vi "Autoliftswitch.vi"() -> ()   [LabVIEW 2017]
uses:
  <vilib>/Rock Robotics/WPI/ThirdParty/Phoenix-LabVIEW/Motor Controller/Controls/CTRE_Phoenix_MotorControl_ControlMode.ctl
  <vilib>/Rock Robotics/WPI/ThirdParty/Phoenix-LabVIEW/Motor Controller/Get/CTRE_Phoenix_MotorController_GetAnalogData.vi
panel:
  out "error out":errorcluster
  in  "error in (no error)":errorcluster
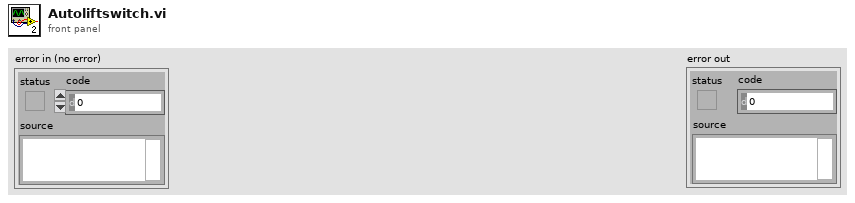
[diagram p1: front panel]
types:
  T1 = typedef "WPI_MotorControlDeviceRef.ctl" = cluster{"DeviceStatus":errorcluster, "Type":T2, "PWM":cluster{"PWM Channel":T3, "DeadBand":T4}, "CAN":cluster{"Device Number":u8, "SetOutput VI Ref":variant, "GetOutput VI Ref":variant, "Enable VI Ref":variant, "Disable VI Ref":variant, "Data":variant}, "Invert":bool, "DIO PWM":cluster{"PWM \"Enable\" Channel":T3, "DIOChannel":T5, "PWM Rate":dbl}}
  T2 = typedef "WPI_MotorControlType.ctl" = enum16{"PWM", "CAN", "DIO PWM"}
  T3 = typedef "FPGA_DIOPWMChannel.ctl" = enum8{"PWM 0", "PWM 1", "PWM 2", "PWM 3", "PWM 4", "PWM 5", "PWM 6", "PWM 7", "PWM 8", "PWM 9", "PWM MXP 0", "PWM MXP 1", "PWM MXP 2", "PWM MXP 3", "PWM MXP 4", "PWM MXP 5", "PWM MXP 6", "PWM MXP 7", "PWM MXP 8", "PWM MXP 9", "Invalid"}
  T4 = typedef "WPI_PWMDeadband.ctl" = cluster{"Name":string, "maxPositivePwm":i32, "minPositivePwm":i32, "centerPwm":i32, "maxNegativePwm":i32, "minNegativePwm":i32, "angularRange":u16}
  T5 = typedef "FPGA_DIOChannel.ctl" = enum8{"DIO 0", "DIO 1", "DIO 2", "DIO 3", "DIO 4", "DIO 5", "DIO 6", "DIO 7", "DIO 8", "DIO 9", "DIO MXP 0", "DIO MXP 1", "DIO MXP 2", "DIO MXP 3", "DIO MXP 4", "DIO MXP 5", "DIO MXP 6", "DIO MXP 7", "DIO MXP 8", "DIO MXP 9", "DIO MXP 10", "DIO MXP 11", "DIO MXP 12", "DIO MXP 13", "DIO MXP 14", "DIO MXP 15", "SPI Port CS1", "SPI Port CS2", "SPI Port CS3", "SPI Port MISO", "SPI Port MOSI", "Invalid"}
  T6 = typedef "CTRE_Phoenix_MotorControl_ControlMode.ctl" = u16
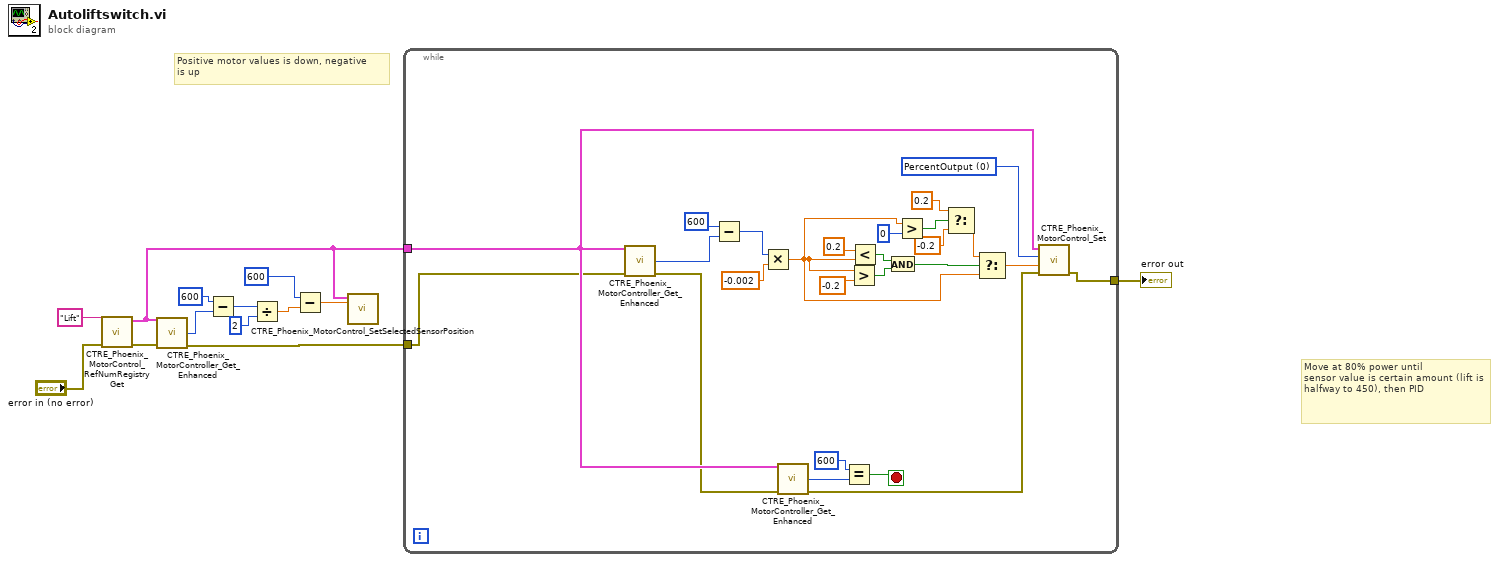
[diagram p0: block diagram]
diagram:
  # "Move at 80% power until\nsensor value is certain amount (lift is halfway to 450), then PID"
  # "Positive motor values is down, negative \nis up"
  n1 = call <vilib>:"CTRE_Phoenix_MotorControl_RefNumRegistryGet.vi"("error in (no error)"="error in (no error)", "refnum name"="Lift") -> ("error out"=w11:errorcluster, "PhoenixMotorControlDevRef"=w2:T1)  [unwired: 8 in]
  n2 = call-poly <vilib>:"CTRE_Phoenix_MotorController_Get_Enhanced.vi"("PhoenixMotorControlDevRef"=w2, "error in"=w11) -> ("AnalogInRaw"=w10:i32, "error out"=w5:errorcluster)  [unwired: 9 in, 3 out]
  n3 = Subtract(x=600, y=w10) -> (x-y=w13:i32)
  n4 = Divide(x=w13, y=2) -> (x/y=w12:dbl)
  n5 = Subtract(x=600, y=w12) -> (x-y=w1:dbl)
  n6 = call <vilib>:"CTRE_Phoenix_MotorControl_SetSelectedSensorPosition.vi"("New Sensor Position"=w1, "PhoenixMotorControlDevRef"=w2) -> ()  [unwired: 8 in, 2 out]
  n7 = while {
    tunnel: w2 -> [w18]
    tunnel: w5 -> [w17]
    tunnel: [w14] -> w3
    stop <- w31 stop-if-true
    w32 = T6 0 items=["PercentOutput"=0, "Position"=1, "Velocity"=2, "Current"=3, "Follower"=5, "MotionProfile"=6, "MotionMagic"=7, "MotionMagicArc"=8, "MotionProfileArc"=10, "Disabled"=15] ("Control Mode")
    n8 = call-poly <vilib>:"CTRE_Phoenix_MotorController_Get_Enhanced.vi"("PhoenixMotorControlDevRef"=w18, "error in"=w17) -> ("AnalogInRaw"=w21:i32, "error out"=w16:errorcluster)  [unwired: 9 in, 3 out]
    n9 = Subtract(x=600, y=w21) -> (x-y=w20:i32)
    n10 = Multiply(x=w20, y=-0.002) -> (x*y=w19:dbl)
    n11 = call-poly <vilib>:"CTRE_Phoenix_MotorController_Get_Enhanced.vi"("PhoenixMotorControlDevRef"=w18, "error in"=w16) -> ("AnalogInRaw"=w30:i32, "error out"=w15:errorcluster)  [unwired: 9 in, 3 out]
    n12 = Equal?(x=600, y=w30) -> (x = y?=w31:bool)
    n13 = Greater?(x=w19, y=-0.2) -> (0:w35:bool)
    n14 = Less?(x=0.2, y=w19) -> (x < y?=w36:bool)
    n15 = And(x=w36, y=w35) -> (x .and. y?=w34:bool)
    n16 = Greater?(x=w19, y=0) -> (0:w27:bool)
    n17 = Select(t=0.2, s=w27, f=-0.2) -> (s? t:f=w28:dbl)
    n18 = Select(t=w28, s=w34, f=w19) -> (s? t:f=w33:dbl)
    n19 = call <vilib>:"CTRE_Phoenix_MotorControl_Set.vi"("error in (no error)"=w15, "Output"=w33, "Control Mode"=w32, "PhoenixMotorControlDevRef"=w18) -> ("error out"=w14:errorcluster)  [unwired: 6 in, 1 out]
  }
  "error out" <- w3
